vi "parseSecurityNode.vi"(11 "read buffer":string) -> (0 "panic button":bool, 1 "temperature (farenheit)":dbl, 2 "node ID":u8, 3 "parse successful?":bool, 4 "motion sensor":bool, 5 "back door":bool, 6 "front door":bool, 7 "garage door":bool)   [LabVIEW 2011]
panel:
  out "siren":bool
  out "motion sensor power":bool
  out "temperature (celsius)":dbl
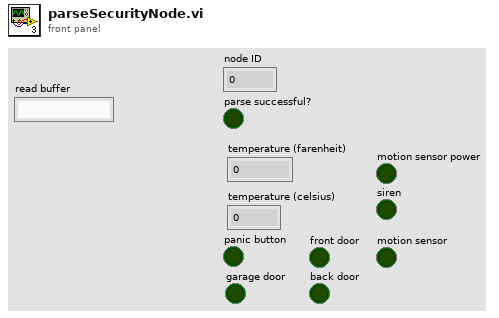
[diagram p1: front panel]
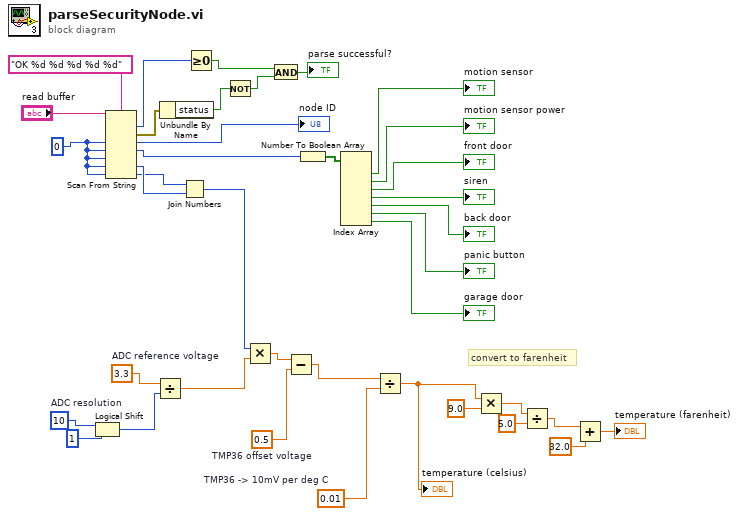
[diagram p0: block diagram]
diagram:
  w22 = 0.01  # TMP36 -> 10mV per deg C
  w24 = 0.5  # TMP36 offset voltage
  w31 = 10  # ADC resolution
  w29 = 3.3  # ADC reference voltage
  w35 = u8 0
  # "convert to farenheit"
  n1 = Logical Shift(y=w31, x=1) -> (x << y=w28:i32)
  n2 = Scan From String(format string="OK %d %d %d %d %d", input string="read buffer", default 1=w35, default 2=w35, default 3=w35, default 4=w35, default 5=w35) -> (offset past scan=w36:u32, error out=w14:errorcluster, output 1=→"node ID":u8, output 2=w9:u8, output 4=w33:u8, output 5=w32:u8)  [unwired: 3 in, 1 out]
  n3 = Divide(x=w29, y=w28) -> (x/y=w26:dbl)
  n4 = Unbundle By Name(w14) -> ("status"=w13:bool)
  n5 = Join Numbers(hi=w32, lo=w33) -> ((hi.lo)=w27:u16)
  n6 = Greater Or Equal To 0?(x=w36) -> (x >= 0?=w12:bool)
  n7 = Not(x=w13) -> (.not. x?=w11:bool)
  n8 = Multiply(x=w27, y=w26) -> (x*y=w25:dbl)
  n9 = And(x=w12, y=w11) -> (x .and. y?=→"parse successful?":bool)
  n10 = Subtract(x=w25, y=w24) -> (x-y=w23:dbl)
  n11 = Number To Boolean Array(number=w9) -> (Boolean array=w8:bool[])
  n12 = Index Array(array=w8) -> (element #1=→"motion sensor":bool, element #2=→"motion sensor power":bool, element #3=→"front door":bool, element #4=→"siren":bool, element #5=→"back door":bool, element #6=→"panic button":bool, element #7=→"garage door":bool)  [unwired: 7 in]
  n13 = Divide(x=w23, y=w22) -> (x/y=w18:dbl)
  "temperature (celsius)" <- w18
  n14 = Multiply(x=w18, y=9.0) -> (x*y=w20:dbl)
  n15 = Divide(x=w20, y=5.0) -> (x/y=w17:dbl)
  n16 = Add(x=w17, y=32.0) -> (x+y=→"temperature (farenheit)":dbl)
